vi "Stop Server.vi"(8 "error in (no error)":errorcluster, 11 "RP Communicator in":refnum<class "RP Communicator.lvclass">) -> (0 "error out":errorcluster, 3 "RP Communicator out":refnum<class "RP Communicator.lvclass">)   [LabVIEW 2024, in "RP Communicator.lvclass"]
uses:
  RP Communicator.lvclass
  RP Communicator.lvclass/RP Communicator.ctl
  RP Command.ctl
  RP Write Command TCP.vi
panel:
  in  "Send \"Connect client\"":bool
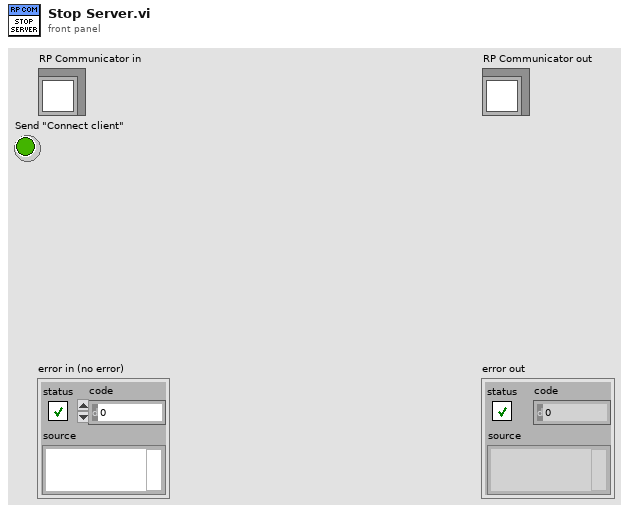
[diagram p1: front panel]
types:
  T1 = typedef "RP Command.ctl" = enum16{"Reset", "Read IDN", "Stop server", "Get status", "Get temperature", "Connect client", "Arm", "Software trigger", "Get whole buffer", "Get chunk", "System call", "Get config", "Set config", "Recieve data", "Recieve Calibartion", "Transmit data"}
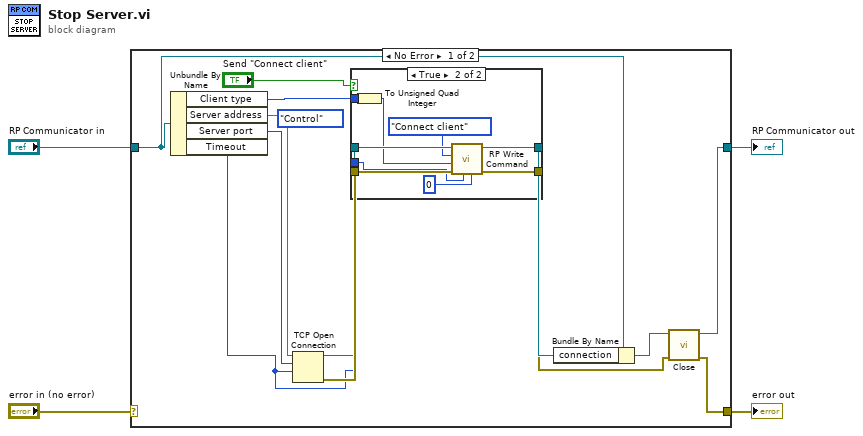
[diagram p0: block diagram]
diagram:
  n1 = case shown="No Error" "error in (no error)" {
    selector: "error in (no error)" -> [_ w30]
    tunnel: [w7 w30] -> w3
    tunnel: [w5 w29] -> w1
    tunnel: "RP Communicator in" -> [w9 w29]
    frame No Error {
      (unwired) enum16{"Control", "Reciever", "Transmitter"}."Control" ("Client type")
      n2 = Unbundle By Name(w9) -> ("Client type"=w13:enum16{"Control", "Reciever", "Transmitter"}, "Server address"=w17:string, "Server port"=w16:u16, "Timeout"=w10:i32)
      n3 = TCP Open Connection(address=w17, remote port or service name=w16, timeout ms (60000)=w10) -> (connection ID=w14:refnum<k5>, error out=w15:errorcluster)  [unwired: 2 in]
      n4 = case shown="True" "Send \"Connect client\"" {
        tunnel: w15 -> [w18 w28]
        tunnel: w14 -> [w19 w27]
        tunnel: w13 -> [_ w25]
        tunnel: [w19 w23] -> w12
        tunnel: [w18 w22] -> w8
        tunnel: w10 -> [_ w21]
        frame False {
        }
        frame True {
          n5 = To Unsigned Quad Integer(1:w25) -> (0:w24:u64)
          n6 = call-poly "RP Write Command.vi"("bytes to read"=0, "timeout ms (25000)"=w21, "Error In"=w28, "Command payload"=w24, "Command number"=RP_Command."Connect client", "connection ID"=w27) -> ("Error Out"=w22:errorcluster, "connection ID out"=w23:refnum<k5>)  [unwired: 2 in, 2 out]
        }
      }
      n7 = Bundle By Name(cluster=w9, "connection"=w12) -> (w6:refnum<class "RP Communicator.lvclass">)
      n8 = call-dynamic "Close.vi"("error in (no error)"=w8, "RP Communicator in"=w6) -> ("error out"=w7:errorcluster, "RP Communicator out"=w5:refnum<class "RP Communicator.lvclass">)  [unwired: 8 in]
    }
    frame Error {
    }
  }
  "error out" <- w3
  "RP Communicator out" <- w1
